vi "Create Stream.vi"(6 "Server Stream":bool, 8 "error in (no error)":errorcluster, 10 "TCP Connection":refnum<k5>, 11 "Websocket Client in":refnum<class "Websocket Client.lvclass">) -> (0 "error out":errorcluster, 3 "Websocket Client out":refnum<class "Websocket Client.lvclass">)   [LabVIEW 2020, in "Stream-Websocket.lvlib" / "Websocket Client.lvclass"]
uses:
  Websocket Client.lvclass
  C:/dev/lv20CE/relink/lv-stream/stream/Endpoint/Endpoint.lvclass
  Websocket Client.lvclass/Websocket Client.ctl
  WebsocketStream/WebsocketStream.lvclass
  C:/dev/lv20CE/relink/lv-stream/stream/Stream/Stream.lvclass
  lv-stream/stream/Endpoint/Endpoint.lvclass
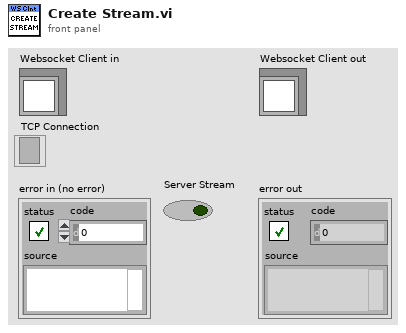
[diagram p1: front panel]
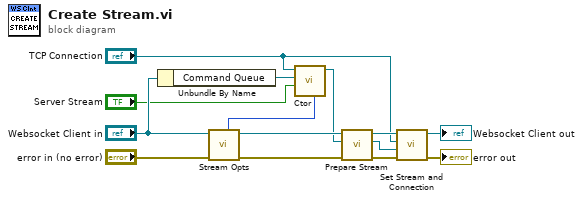
[diagram p0: block diagram]
diagram:
  n1 = Unbundle By Name("Websocket Client in") -> ("Command Queue"=w14:refnum<queue>)
  n2 = call "Stream Opts.vi"("error in (no error)"="error in (no error)", "Websocket Client in"="Websocket Client in") -> ("error out"=w10:errorcluster, "Websocket Client out"=w12:refnum<class "Websocket Client.lvclass">, "Timeout ms"=w13:i32)  [unwired: 7 in]
  n3 = call "Ctor.vi"("Timeout ms"=w13, "Server Stream"="Server Stream", "Command Queue"=w14, "TCP Connection"="TCP Connection") -> ("WebsocketStream out"=w11:refnum<class "WebsocketStream.lvclass">)  [unwired: 6 in, 1 out]
  n4 = call "Prepare Stream.vi"("error in (no error)"=w10, "Stream In"=w11, "Endpoint in"=w12) -> ("error out"=w6:errorcluster, "Stream"=w8:refnum<class "WebsocketStream.lvclass">, "Endpoint out"=w9:refnum<class "Websocket Client.lvclass">)  [unwired: 6 in]
  n5 = call "Set Stream and Connection.vi"("error in (no error)"=w6, "Stream"=w8, "TCP Connection"="TCP Connection", "Websocket Client in"=w9) -> ("error out"=→"error out":errorcluster, "Websocket Client out"=→"Websocket Client out":refnum<class "Websocket Client.lvclass">)  [unwired: 6 in]
